vi "Set URI String.vi"(8 "error in (no error)":errorcluster, 10 "URI String":string, 11 "URI in":refnum<class "URI.lvclass">) -> (0 "error out":errorcluster, 3 "URI out":refnum<class "URI.lvclass">)   [LabVIEW 2020, in "IO.lvlib" / "URI.lvclass"]
uses:
  URI.lvclass
  URI.lvclass/URI.ctl
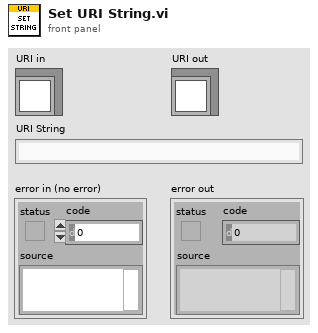
[diagram p1: front panel]
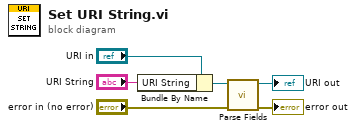
[diagram p0: block diagram]
diagram:
  n1 = Bundle By Name(cluster="URI in", "URI String"="URI String") -> (w5:refnum<class "URI.lvclass">)
  n2 = call "Parse Fields.vi"("error in (no error)"="error in (no error)", "URI in"=w5) -> ("error out"=→"error out":errorcluster, "URI out"=→"URI out":refnum<class "URI.lvclass">)  [unwired: 8 in]
